vi "set_x.vi"(0 "HB_Simple":refnum<class "HB_Simple.lvclass">, 2 "x":dbl, 5 "error in (no error)":errorcluster) -> (14 "dup HB_Simple":refnum<class "HB_Simple.lvclass">, 19 "error out":errorcluster)   [LabVIEW 2009, in "HB_BaseClass_Examples.lvlib" / "HB_Simple.lvclass"]
doc: "Write value of x."
uses:
  HB_Simple.lvclass
  HB_Simple.lvclass/HB_Simple.ctl
  lib.lib/HGF_LVC/HGF_BaseClasses/HGF_TriggeredEvent/HGF_TriggeredEvent.lvclass
  lib.lib/HGF_LVC/HGF_BaseClasses/HGF_PVPublisher/HGF_PVPublisher.lvclass
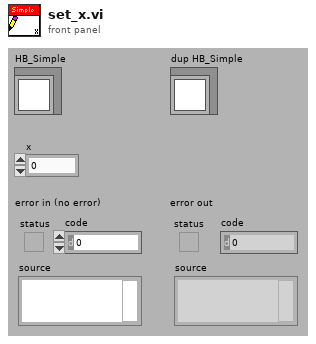
[diagram p1: front panel]
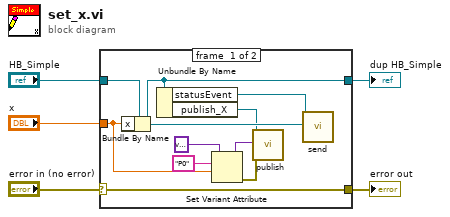
[diagram p0: block diagram]
diagram:
  n1 = case shown="No Error" "error in (no error)" {
    selector: "error in (no error)" -> [w15 w16]
    tunnel: [w15 w16] -> w4
    tunnel: [w12 w17] -> w2
    tunnel: "HB_Simple" -> [w14 w17]
    tunnel: "x" -> [w6 _]
    frame #0 {
      n2 = Bundle By Name(cluster=w14, "x"=w6) -> (w12:refnum<class "HB_Simple.lvclass">)
      n3 = Unbundle By Name(w12) -> ("statusEvent"=w13:refnum<class "HGF_TriggeredEvent.lvclass">, "publish_X"=w7:refnum<class "HGF_PVPublisher.lvclass">)
      n4 = Set Variant Attribute(Variant=variant ("variant"), name="P0", value=w6) -> (Variant out=w10:variant, error out=w11:errorcluster)  [unwired: 1 in, 1 out]
      n5 = call-dynamic "publish.vi"("HGF_PVPublisher"=w7, "data"=w10, "error in (no error)"=w11) -> ()  [unwired: 2 in, 15 out]
      n6 = call-dynamic "send.vi"("HGF_Event"=w13, "Object"=w12) -> ()  [unwired: 3 in, 15 out]
    }
    frame #1 {
    }
  }
  "error out" <- w4
  "dup HB_Simple" <- w2
